vi "PIDPressure1.vi"() -> ()   [LabVIEW 2015]
uses:
  <vilib>/DAQmx/write.llb/DAQmx Write (Analog DBL 1Chan 1Samp).vi
  <vilib>/Analysis/baseanly.llb/Mean (DBL).vi
  <vilib>/DAQmx/read.llb/DAQmx Read (Analog 1D Wfm NChan NSamp).vi
  <vilib>/DAQmx/miscellaneous.llb/DAQmx Fill In Error Info.vi
  <vilib>/addons/control/pid/NI_PID_autopid.lvlib
  <vilib>/Analysis/NI_AALBase.lvlib
panel:
  out "Loop 1":i32
  out "Loop 2":i32
  in  "Voltage setting":dbl format="%#_13g"
  in  "Manual Control":bool
  out "Control Value":dbl
  in  "setpoint in Bar":dbl format="%#.5f"
  in  "reinitialize? (F)":bool
  in  "autotune? (F)":bool
  out "PID gains out":T1={"proportional gain (Kc)"=1.0, "integral time (Ti, min)"=0.01, "derivative time (Td, min)"=0.0} {"derivative time (Td, min)" format="%.3f"; "integral time (Ti, min)" format="%.3f"; "proportional gain (Kc)" format="%.3f"}
  in  "PID gains":T1={"proportional gain (Kc)"=1.0, "integral time (Ti, min)"=0.01, "derivative time (Td, min)"=0.0} {"derivative time (Td, min)" format="%.3f"; "integral time (Ti, min)" format="%.3f"; "proportional gain (Kc)" format="%.3f"}
  in  "autotuning parameters":T2={"controller type"=1, "relay cycles"=3, "relay amplitude"=1.0, "control specification"=2, "PV noise level"=0.1} {"PV noise level" format="%.2f"; "control specification" items=["normal", "fast", "slow"]; "relay amplitude" format="%.2f"; "controller type" items=["PID", "PI", "P"]}
  in  "stop":bool
  out "Pressure Chart 2":dbl(graph)
  out "Voltage":dbl(graph)
  out "Pressure":dbl format="%#.3g"
  out "Voltage Reading(pressure)":dbl format="%#_13g"
  # "51.12139\n\n0.044676"
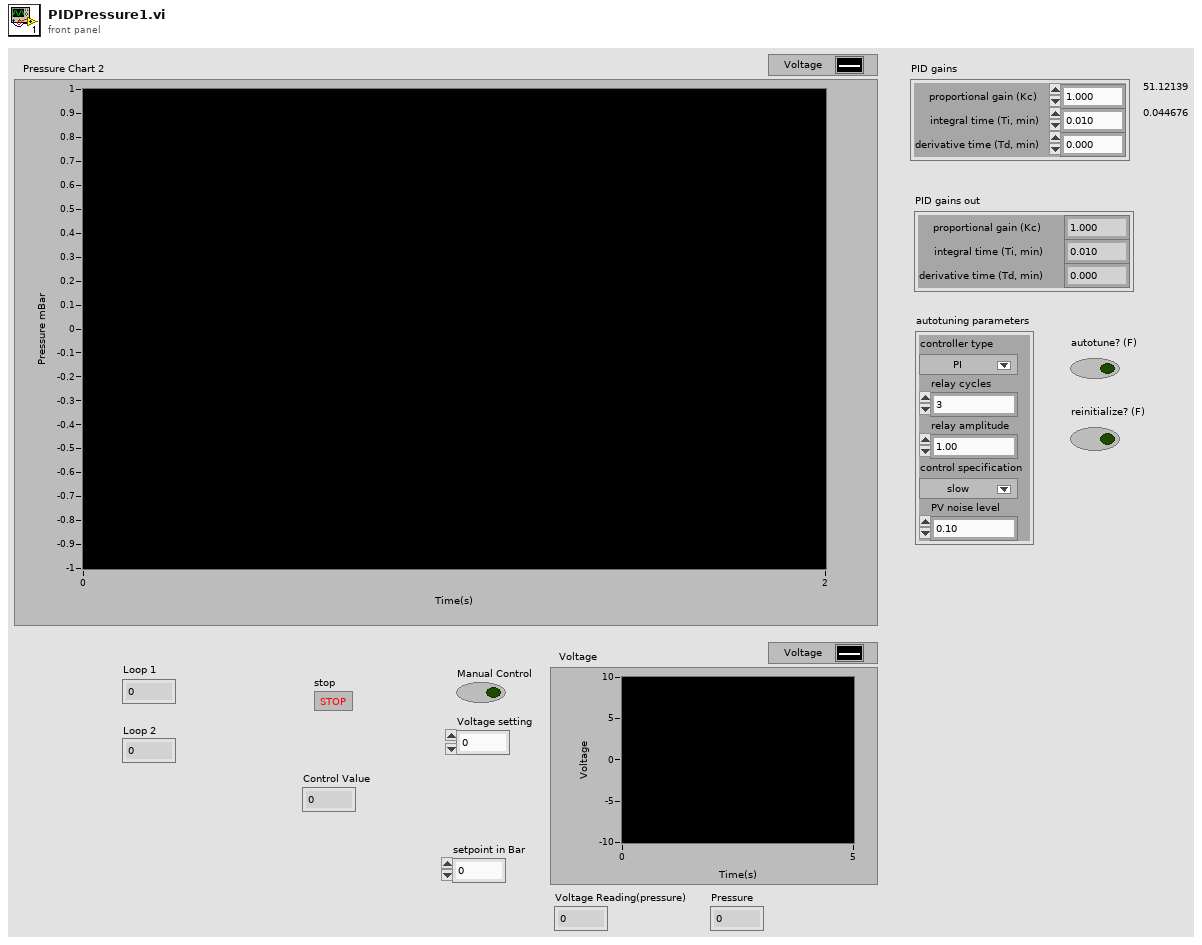
[diagram p1: front panel]
types:
  T1 = cluster{"proportional gain (Kc)":dbl, "integral time (Ti, min)":dbl, "derivative time (Td, min)":dbl}
  T2 = cluster{"controller type":u16, "relay cycles":i32, "relay amplitude":dbl, "control specification":u16, "PV noise level":dbl}
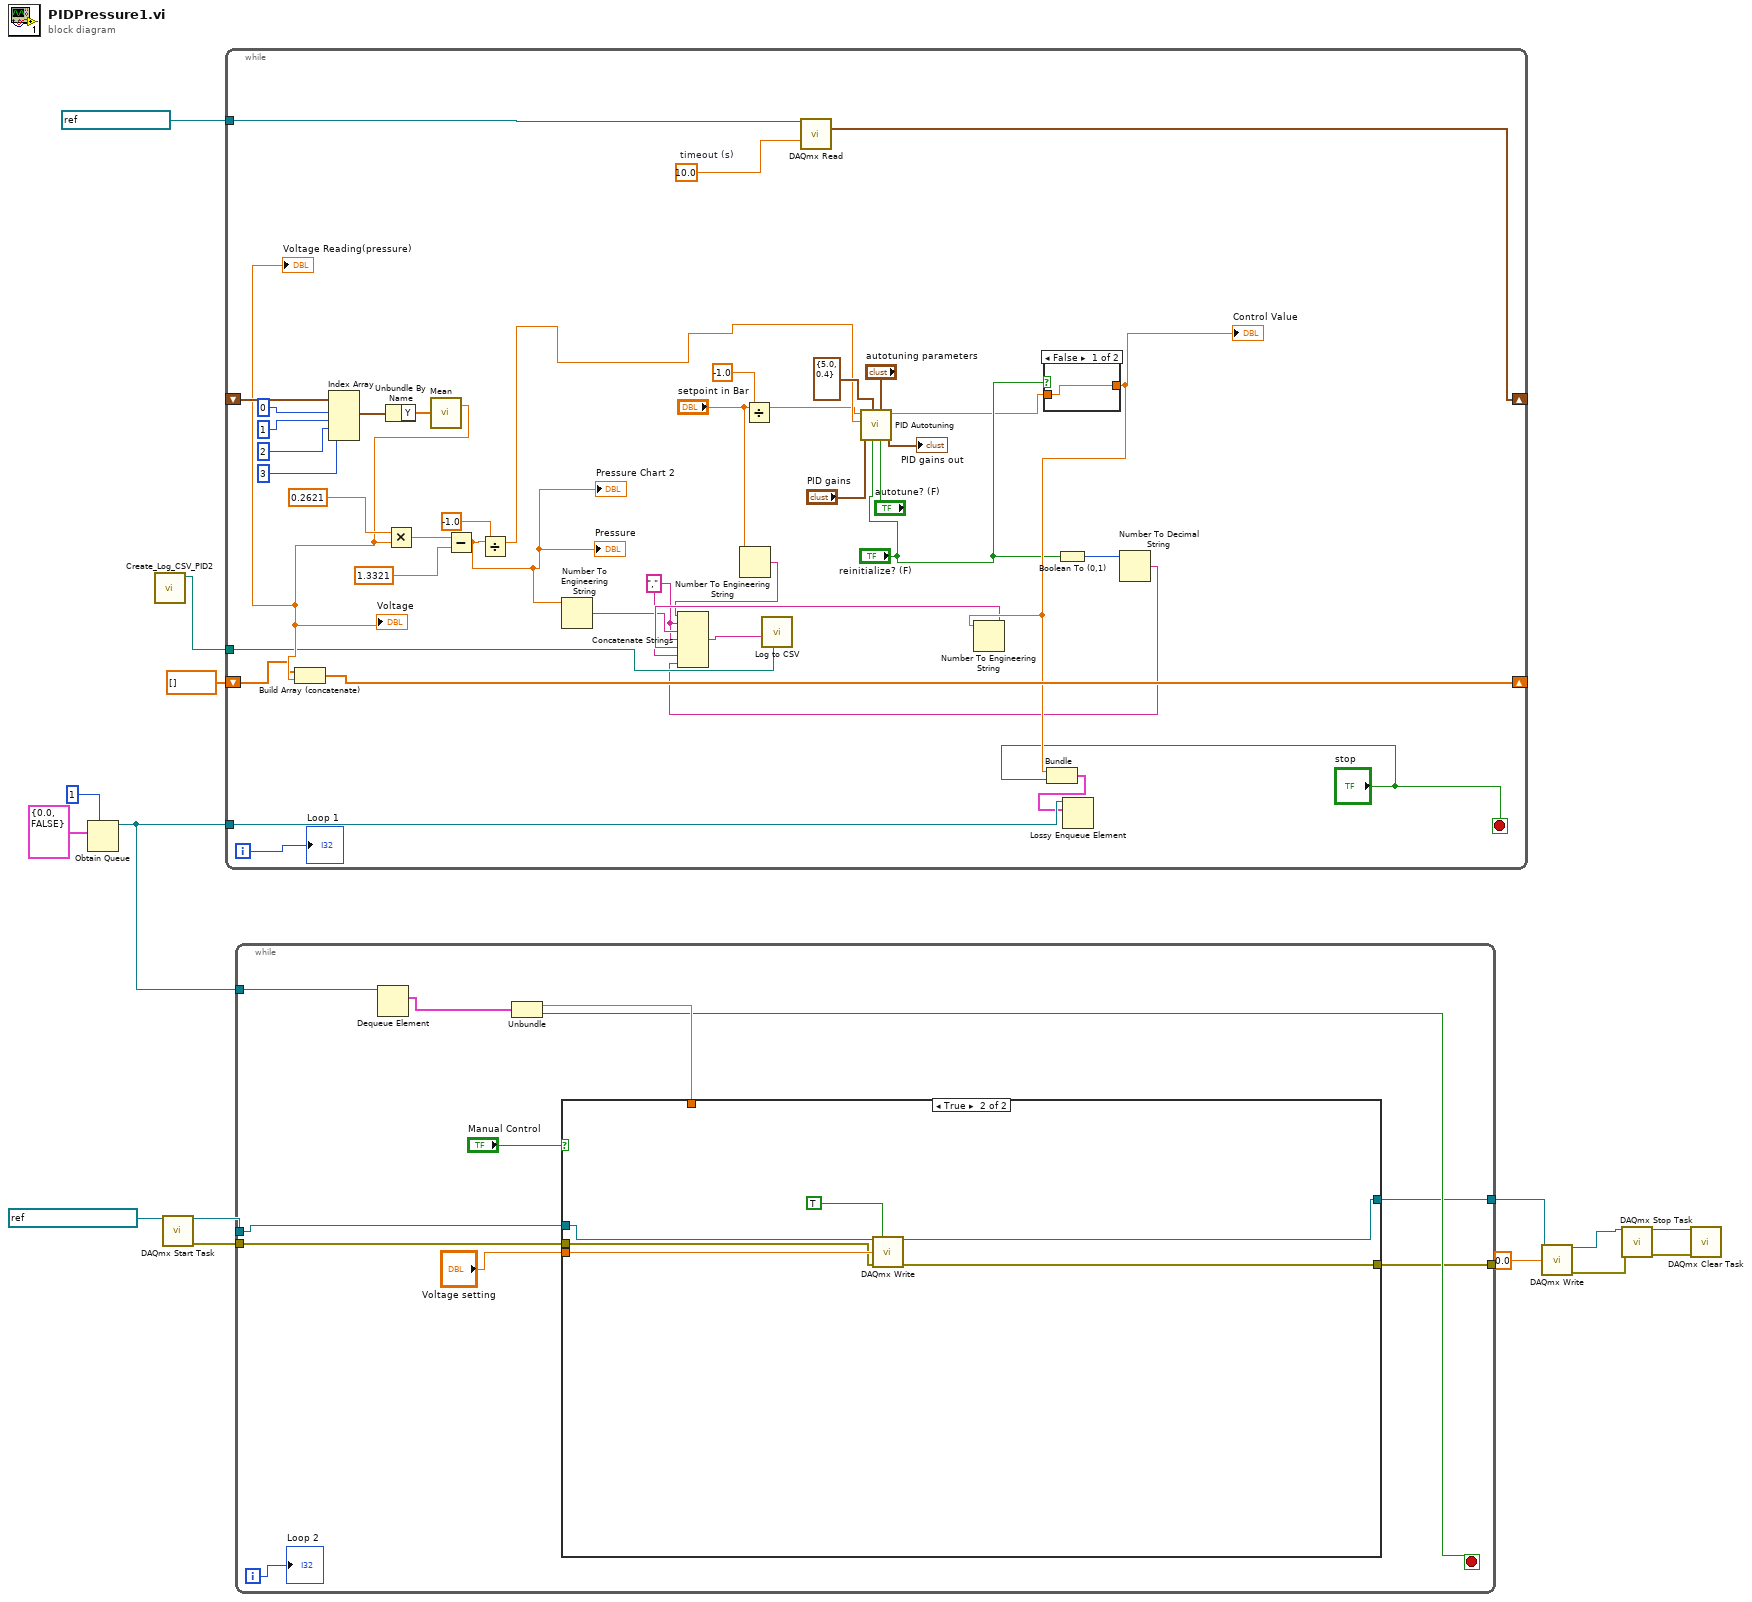
[diagram p0: block diagram]
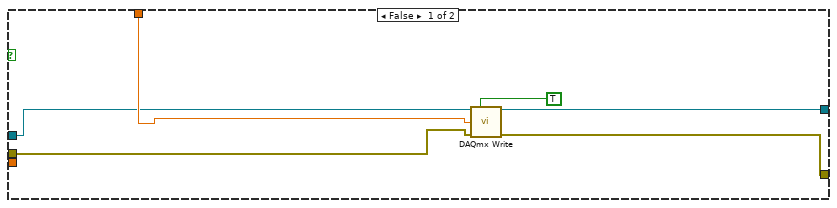
[diagram p2: hidden frame]
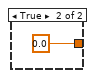
[diagram p3: hidden frame]
diagram:
  n1 = Obtain Queue(max queue size (-1, unlimited)=1, element data type=cluster{dbl, bool} {0.0, FALSE}) -> (queue out=w13:refnum<queue>)  [unwired: 3 in, 2 out]
  n2 = call "Create_Log_CSV_PID2.vi"() -> ("path"=w9:path)  [unwired: 11 in]
  n3 = call <vilib>:"DAQmx Start Task.vi"("task/channels in"=refnum<k21> "MyVoltageOutTask") -> ("task out"=w8:refnum<k21>, "error out"=w7:errorcluster)  [unwired: 13 in]
  n4 = while {
    tunnel: refnum<k21> "MyVoltageTask" -> [w53]
    shift-right: [w47] -> _
    shift-left: _ -> [w40]
    tunnel: w13 -> [w46]
    shift-right: [w35] -> _
    shift-left: dbl[] [] -> [w36]
    tunnel: w9 -> [w29]
    i -> [w21]
    stop <- "stop" stop-if-true
    w24 = ","
    w57 = 10.0  # timeout (s)
    n5 = Index Array(array=w40, index #1=0 ("index"), index #2=1 ("index"), index #3=2 ("index"), index #4=3 ("index")) -> (element #1=w39:waveform(dbl))  [unwired: 3 out]
    n6 = Unbundle By Name(w39) -> ("Y"=w38:dbl[])
    n7 = call-poly <vilib>:"Mean.vi"("X"=w38) -> ("mean"=w37:dbl)  [unwired: 1 out]
    "Voltage Reading(pressure)" <- w37
    "Voltage" <- w37
    n8 = Build Array (concatenate)(w36, w37) -> (w35:dbl[])
    n9 = Multiply(x=0.2621, y=w37) -> (x*y=w55:dbl)
    n10 = Subtract(x=w55, y=1.3321) -> (x-y=w33:dbl)
    "Pressure" <- w33
    "Pressure Chart 2" <- w33
    n11 = Divide(x=w33, y=-1.0) -> (x/y=w19:dbl)
    n12 = Number To Engineering String(4:w33) -> (0:w28:string)  [unwired: 3 in]
    n13 = Number To Engineering String(4:"setpoint in Bar") -> (0:w27:string)  [unwired: 3 in]
    n14 = Divide(x="setpoint in Bar", y=-1.0) -> (x/y=w18:dbl)
    n15 = call-poly <vilib>:"DAQmx Read.vi"("task/channels in"=w53, "timeout"=w57) -> ("data"=w47:waveform(dbl)[])  [unwired: 11 in, 2 out]
    n16 = call <vilib>:"PID Autotuning.vi"("autotune? (F)"="autotune? (F)", "autotuning parameters"="autotuning parameters", "reinitialize? (F)"="reinitialize? (F)", "output range"=cluster{"output high":dbl, "output low":dbl} {"output high"=5.0, "output low"=0.4}, "PID gains"="PID gains", "process variable"=w19, "setpoint"=w18) -> ("PID gains out"=→"PID gains out":T1, "output"=w16:dbl)  [unwired: 1 in, 2 out]
    n17 = case shown="False" "reinitialize? (F)" {
      tunnel: [w58 0.0] -> w32
      tunnel: w16 -> [w58 _]
      frame False {
      }
      frame True {
      }
    }
    "Control Value" <- w32
    n18 = Number To Engineering String(4:w32) -> (0:w31:string)  [unwired: 3 in]
    n19 = Bundle("output"=w32, "stop"="stop") -> (w45:cluster{"output":dbl, "stop":bool})  [unwired: 1 in]
    n20 = Boolean To (0,1)(Boolean="reinitialize? (F)") -> (0, 1=w25:i16)
    n21 = Lossy Enqueue Element(queue=w46, element=w45) -> ()  [unwired: 1 in, 4 out]
    n22 = Number To Decimal String(number=w25) -> (decimal integer string=w23:string)  [unwired: 1 in]
    n23 = Concatenate Strings(w27, w24, w28, w24, w31, w24, w23) -> (w30:string)
    n24 = call "Log to CSV.vi"("Data Str"=w30, "Path"=w29) -> ()  [unwired: 5 in, 1 out]
    "Loop 1" <- w21
  }
  n25 = while {
    tunnel: w13 -> [w70]
    tunnel: w8 -> [w68]
    tunnel: [w62] -> w5
    tunnel: w7 -> [w61]
    tunnel: [w60] -> _
    i -> [w64]
    stop <- w63 stop-if-true
    n26 = Dequeue Element(queue=w70) -> (element=w67:cluster{dbl, bool})  [unwired: 2 in, 3 out]
    n27 = Unbundle(w67) -> (w66:dbl, w63:bool)
    n28 = case shown="True" "Manual Control" {
      tunnel: w68 -> [w74 w81]
      tunnel: w66 -> [w75 _]
      tunnel: "Voltage setting" -> [_ w80]
      tunnel: [w73 w79] -> w62
      tunnel: w61 -> [w72 w78]
      tunnel: [w71 w77] -> w60
      frame False {
        n29 = call-poly <vilib>:"DAQmx Write.vi"("task/channels in"=w74, "auto start"=TRUE, "data"=w75, "error in"=w72) -> ("task out"=w73:refnum<k21>, "error out"=w71:errorcluster)  [unwired: 9 in, 1 out]
      }
      frame True {
        n30 = call-poly <vilib>:"DAQmx Write.vi"("task/channels in"=w81, "auto start"=TRUE, "data"=w80, "error in"=w78) -> ("task out"=w79:refnum<k21>, "error out"=w77:errorcluster)  [unwired: 9 in, 1 out]
      }
    }
    "Loop 2" <- w64
  }
  n31 = call-poly <vilib>:"DAQmx Write.vi"("task/channels in"=w5, "data"=0.0) -> ("task out"=w4:refnum<k21>, "error out"=w3:errorcluster)  [unwired: 11 in, 1 out]
  n32 = call <vilib>:"DAQmx Stop Task.vi"("task/channels in"=w4, "error in"=w3) -> ("task out"=w6:refnum<k21>, "error out"=w2:errorcluster)  [unwired: 12 in]
  n33 = call <vilib>:"DAQmx Clear Task.vi"("task in"=w6, "error in"=w2) -> ()  [unwired: 13 in, 1 out]
